vi "FXP2Volt.vi"(11 "Input (Int)":fxp<+,22,12>) -> (3 "Output (FXP)":fxp<+,25,3>)   [LabVIEW 2017, in "FPGA functions.lvlib"]
doc: "Convert 12-bit unsigned integer + decimals due to oversampling and averaging (FXP) into Voltage representation (FXP +25,3) between 0 to 5 V."
uses:
  FPGA functions.lvlib
  <vilib>/Platform/TimedLoop/XDataNode/XDataNode.xnode
  <vilib>/Platform/TimedLoop/XDataNode/nitl_modes.ctl
  <vilib>/Platform/TimedLoop/XDataNode/XDNodeRunTimeDep.lvlib
  <vilib>/Platform/TimedLoop/XDataNode/wakeup.ctl
  <vilib>/Platform/TimedLoop/XDataNode/timing_clust.ctl
  <vilib>/rvi/FXPMathLib/FxpMul/XNode/nifxpmath_Multiplier.xnode
  <vilib>/rvi/FXPMathLib/sim/FxpSim.dll
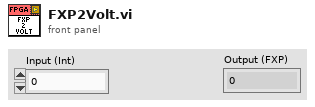
[diagram p1: front panel]
types:
  T1 = typedef "XDNodeRunTimeDep.lvlib/timing_clust.ctl" = cluster{"Expected End [f-1]":u64, "Actual End [f-1]":u64, "Finished Late? [f-1]":bool, "Expected End [i-1]":u64, "Actual End [i-1]":u64, "Finished Late? [i-1]":bool, "Expected Start [i]":u64, "Actual Start [i]":u64, "Expected Start [f]":u64, "Actual Start [f]":u64, "Source Name":string, "Structure Name":string, "Period":i64, "Deadline":i64, "Offset":i64, "Start":i64, "Priority":i32, "Timeout":i32, "Mode":T2, "Wakeup Reason":T3, "Error":errorcluster, "Source Type":string, "Secondary Source Type":string, "Global End Time":u64, "Global Start Time":u64, "Frame Duration":u64, "Iteration Duration":u64, "Assigned CPU":i32, "I/O Scan Engine Mode":u32}
  T2 = typedef "XDNodeRunTimeDep.lvlib/nitl_modes.ctl" = enum32{"No Change", "Process missed periods, maintain original phase", "Discard missed periods, maintain original phase", "Process missed periods, ignore original phase", "Discard missed periods, ignore original phase"}
  T3 = typedef "XDNodeRunTimeDep.lvlib/wakeup.ctl" = enum32{"Normal", "Aborted", "Asynchronous wakeup", "Timing source error", "Timed loop error", "Timeout"}
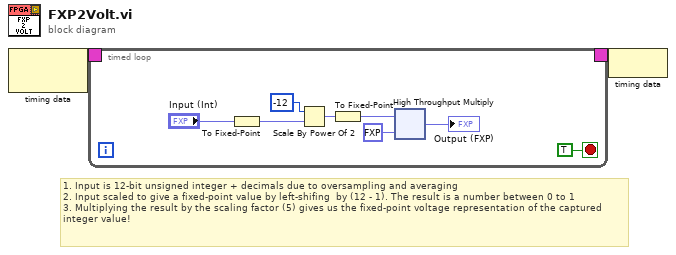
[diagram p0: block diagram]
diagram:
  # "1. Input is 12-bit unsigned integer + decimals due to oversampling and averaging\n2. Input scaled to give a fixed-point value by left-shifing  by (12 - 1). The result is a number between 0 to 1\n3. Multiplying the result by the scaling factor (5) gives us the fixed-point voltage representation of the captured integer value!"
  n1 = node-c288() -> (w2:T1)  [unwired: 1 in]
  n2 = timed-loop {
    timing: w2 -> [_]
    timing-out: [_] -> w1
    stop <- TRUE stop-if-true
    n3 = To Fixed-Point(number="Input (Int)") -> (fixed-point=w10:fxp<+,32,12>)  [unwired: 1 in]
    n4 = Scale By Power Of 2(n=i16 -12, x=w10) -> (x*2^n=w8:fxp<+,32,12>)
    n5 = To Fixed-Point(number=w8) -> (fixed-point=w7:fxp<+,22,0>)  [unwired: 1 in]
    n6 = xnode "High Throughput Multiply"("x"=w7, "y"=fxp<+,3,3> 5.0 ("Multiplier")) -> ("x*y"=→"Output (FXP)":fxp<+,25,3>)
  }
  n7 = node-c288(w1) -> ()
